vi "(SubVI) Acquire precise position_YCC.vi"(4 "Axis":u32=1, 5 "record time (s)":dbl=0.1) -> (1 "precise current position (um)":dbl format="%0.5f")   [LabVIEW 2014]
uses:
  (Global) Current handle and LaserPower_YCC.vi
  <vilib>/Analysis/NI_AALBase.lvlib
  MCL-dll-Labview 32-bit/Madlib.dll
panel:
  out "standard deviation (nm)":dbl format="%0.2f"
  out "Data point":dbl
  out "Acq. rate (Hz)":dbl
  in  "ADC Rate (ms)":T1(ring)=enum."1000 Hz"
  # "3 -> 267us, 4 -> 500us , 5 -> 1ms , 6 -> 2ms, 7 -> 10ms , 8 -> 17ms , 9 -> 20ms"
  # "for 16bit\n5 ms to 0.1 ms\n(200Hz to 10k Hz)"
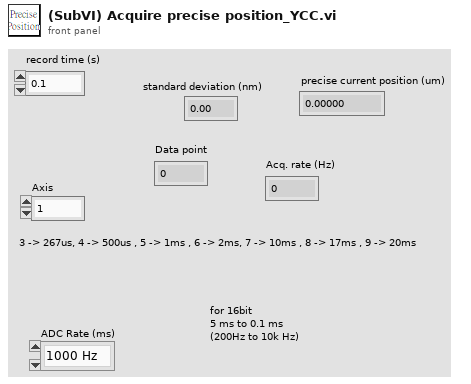
[diagram p1: front panel]
types:
  T1 = enum16{"50 Hz", "60 Hz", "100 Hz", "500 Hz", "1000 Hz", "2000 Hz", "3750 Hz"}
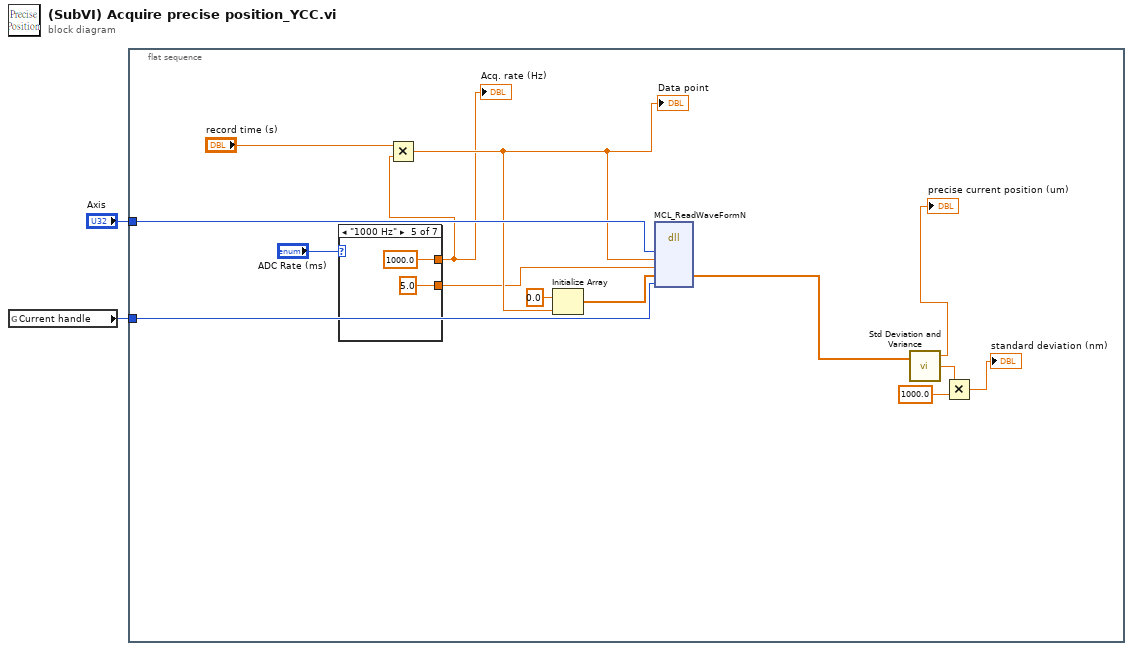
[diagram p0: block diagram]
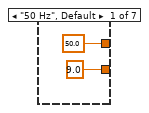
[diagram p2: hidden frame]
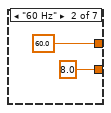
[diagram p3: hidden frame]
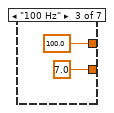
[diagram p4: hidden frame]
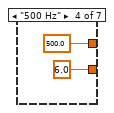
[diagram p5: hidden frame]
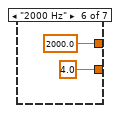
[diagram p6: hidden frame]
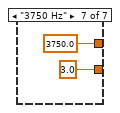
[diagram p7: hidden frame]
diagram:
  n1 = global read "(Global) Current handle and LaserPower_YCC.vi" "Current handle"() -> (w1:i32)
  n2 = flat-sequence {
    tunnel: "Axis" -> [w15]
    tunnel: w1 -> [w14]
    frame #0 {
      n3 = case shown="\"1000 Hz\"" "ADC Rate (ms)" {
        tunnel: [9.0 8.0 7.0 6.0 5.0 4.0 3.0] -> w4
        tunnel: [50.0 60.0 100.0 500.0 1000.0 2000.0 3750.0] -> w5
        frame "50 Hz", Default {
        }
        frame "60 Hz" {
        }
        frame "100 Hz" {
        }
        frame "500 Hz" {
        }
        frame "1000 Hz" {
        }
        frame "2000 Hz" {
        }
        frame "3750 Hz" {
        }
      }
      "Acq. rate (Hz)" <- w5
      n4 = Multiply(x="record time (s)", y=w5) -> (x*y=w7:dbl)
      "Data point" <- w7
      n5 = Initialize Array "Initialize Array"(0.0 ("element"), w7) -> (w9:dbl[])
      n6 = dll-call lib="C:/Users/OT-hwlab/Desktop/YCC's OT/Main-Stage-Based/SubVI-Stage-Based/MCL-dll-Labview 32-bit/MADLib.dll" fn="MCL_ReadWaveFormN"("axis"=w15, "DataPoints"=w7, "milliseconds"=w4, "waveform"=w9, "handle"=w14) -> ("waveform"=w13:dbl[])  [unwired: 8 in, 2 out]
      n7 = call <vilib>:"Std Deviation and Variance.vi"("X"=w13) -> ("mean"=→"precise current position (um)":dbl, "standard deviation"=w12:dbl)  [unwired: 1 in, 1 out]
      n8 = Multiply(x=w12, y=1000.0) -> (x*y=→"standard deviation (nm)":dbl)
    }
  }
